vi "Initialize.vi"(8 "error in (no error)":errorcluster, 11 "HtmlReportPlugin in":refnum<class "HtmlReportPlugin.lvclass">) -> (0 "error out":errorcluster, 3 "HtmlReportPlugin out":refnum<class "HtmlReportPlugin.lvclass">)   [LabVIEW 2015, in "HtmlReportPlugin.lvclass"]
uses:
  HtmlReportPlugin.lvclass
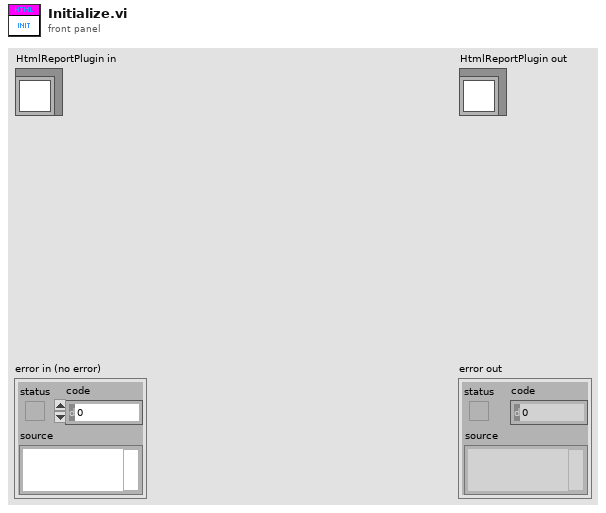
[diagram p1: front panel]
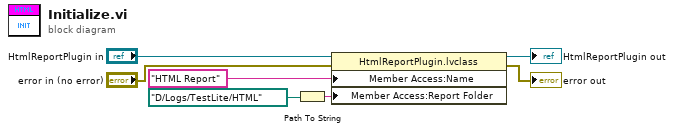
[diagram p0: block diagram]
diagram:
  n1 = Path To String(path=path "D:/Logs/TestLite/HTML" ("Report Folder")) -> (string=w5:string)
  n2 = property class="HtmlReportPlugin.lvclass"(reference="HtmlReportPlugin in", error in="error in (no error)", "Member Access:Name"="HTML Report" ("Name"), "Member Access:Report Folder"=w5) -> (reference out=→"HtmlReportPlugin out":refnum<class "HtmlReportPlugin.lvclass">, error out=→"error out":errorcluster)
